vi "Artificial Strip Chart.vi"() -> ()   [LabVIEW 2023]
doc: "Uses the Plot XY VI to create an XY strip chart in a picture indicator. Because you cannot scroll an arbitrary region of a picture, the VI maintains a limited history of points, and draws them as a graph with each update."
panel:
  in  "Stop":bool
  out "2D Picture":picture
  # "Overview: Uses the Plot XY VI to create an XY strip chart in a picture indicator. \nInstructions:\n1. Run the VI.\n2. Click Stop to stop the VI."
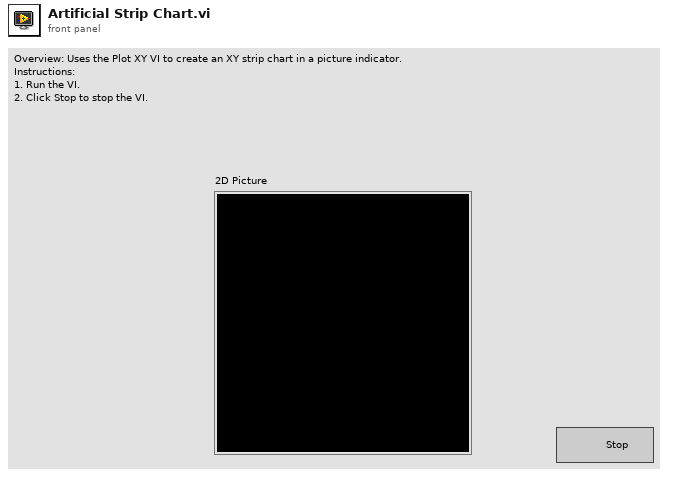
[diagram p1: front panel]
types:
  T1 = cluster{"Initial X Value":dbl, "Initial X Value":dbl}
  T2 = cluster{"Initial X Value":dbl, "Initial X Value":dbl}[]
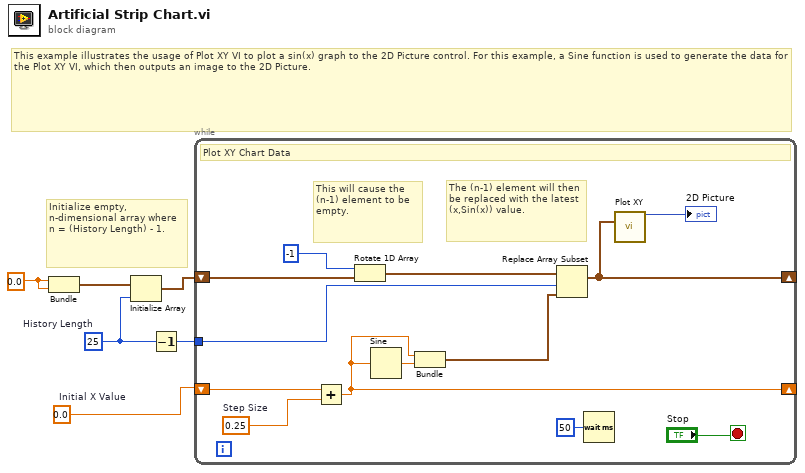
[diagram p0: block diagram]
diagram:
  w4 = 0.0 ("Initial X Value")
  w5 = 0.0  # Initial X Value
  w2 = 25  # History Length
  # "This example illustrates the usage of Plot XY VI to plot a sin(x) graph to the 2D Picture control. For this example, a Sine function is used to generate the data for the Plot XY VI, which then outputs an image to the 2D Picture."
  # "Initialize empty, n-dimensional array where n = (History Length) - 1."
  n1 = Bundle("Initial X Value"=w4, "Initial X Value"=w4) -> (w3:T1)  [unwired: 1 in]
  n2 = Initialize Array(w3, w2) -> (w1:T2)
  n3 = Decrement(x=w2) -> (x-1=w6:i32)
  n4 = while {
    shift-right: [w13] -> _
    shift-left: w1 -> [w18]
    tunnel: w6 -> [w16]
    shift-right: [w12] -> _
    shift-left: w5 -> [w14]
    stop <- "Stop" stop-if-true
    w7 = 0.25  # Step Size
    # "The (n-1) element will then be replaced with the latest (x,Sin(x)) value."
    # "This will cause the (n-1) element to be empty."
    # "Plot XY Chart Data"
    n5 = Add(x=w14, y=w7) -> (x+y=w12:dbl)
    n6 = Rotate 1D Array(1:w18, 2:-1) -> (0:w8:T2)
    n7 = Sine(x=w12) -> (sin(x)=w15:dbl)
    n8 = Bundle(w12, w15) -> (w9:cluster{dbl, dbl})  [unwired: 1 in]
    n9 = Replace Array Subset(array=w8, new element=w9, index=w16) -> (w13:T2)
    n10 = Wait (ms)(milliseconds to wait=u32 50 ("millisecond multiple")) -> ()  [unwired: 1 out]
    n11 = call <vilib>:"Plot XY.vi"("data"=w13) -> ("new picture"=→"2D Picture":picture)  [unwired: 14 in]
  }
